vi "SEND_WIFI_DETAILS.vi"(8 "error in (no error)":errorcluster, 11 "Message":T1={"Payload Size"=0, "Sequence Number"=0, "Sensor Type"=enum."APP", "Message Types"=enum."SEND_LOG_FILE_SIZE", "Data"=[]}) -> (0 "error out":errorcluster, 3 "Current Measurments (csv string)":string)   [LabVIEW 2019]
uses:
  Typedefs/Message.ctl
  Typedefs/Sensor Types.ctl
  Typedefs/Message Types.ctl
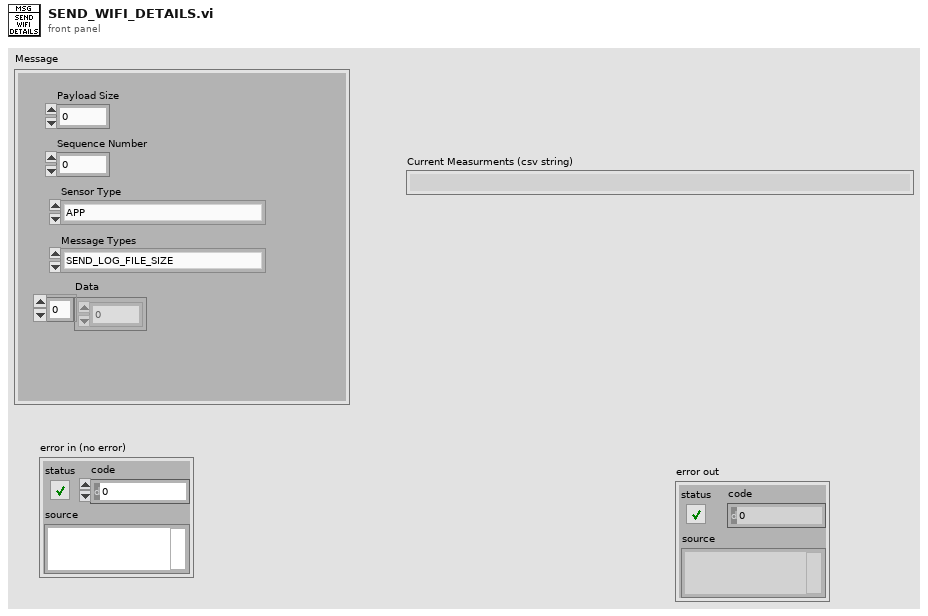
[diagram p1: front panel]
types:
  T1 = typedef "Message.ctl" = cluster{"Payload Size":u8, "Sequence Number":u8, "Sensor Type":T2, "Message Types":T3, "Data":u8[]}
  T2 = typedef "Sensor Types.ctl" = enum16{"APP", "TURBIDITY", "PH"}
  T3 = typedef "Message Types.ctl" = enum16{"HEART_BEAT", "CONNECT", "GET_CURRENT_MEASUREMENTS", "GET_LOG_FILE", "SEND_LOG_FILE_SIZE", "SEND_LOG_FILE_CHUNK", "GET_LOGGING_PERIOD", "SET_LOGGING_PERIOD", "SEND_SD_CARD_INFO", "GET_LOGS_LIST", "SEND_LOG_FILE_NAME", "SEND_LOGGING_PERIOD", "GET_RTC_TIME", "SET_RTC_TIME", "SEND_RTC_TIME", "SEND_CURRENT_MEASUREMENTS", "DELETE_LOG_FILE", "GET_SD_CARD_INFO", "GET_BATTERY_INFO", "SEND_BATTERY_INFO", "GET_LOG_FILE_SIZE", "SET_WIFI_SSID", "SET_WIFI_PASSWORD", "GET_WIFI_DETAILS", "SEND_WIFI_DETAILS", "ERROR_MSG"}
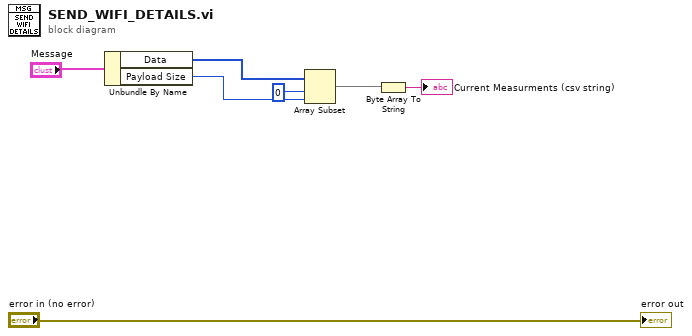
[diagram p0: block diagram]
diagram:
  n1 = Unbundle By Name("Message") -> ("Data"=w3:u8[], "Payload Size"=w2:u8)
  n2 = Array Subset(array=w3, index=0, length=w2) -> (w1:u8[])
  n3 = Byte Array To String(unsigned byte array=w1) -> (string=→"Current Measurments (csv string)":string)
  "error out" <- "error in (no error)"
